vi "Digitizer Analyze_SNRDCOffset.vi"(6 "frequency range":T1={"start frequency"=-1.0, "stop frequency"=-1.0}, 7 "Pins":string[](array[string])=["Xout"], 8 "error in":errorcluster, 9 "Published Data Id":string[](array[string]), 10 "Waveform Data In":waveform(dbl)[](array[waveform])=[{"t0"=timestamp(3637030365.2340937 s since 1904-01-01), "dt"=3.3333333333333334e-08, "Y"=array[5343 elements]}, {"t0"=timestamp(3637030365.2340937 s since 1904-01-01), "dt"=3.3333333333333334e-08, "Y"=array[5343 elements]}], 11 "Semiconductor Module Context":T2) -> (0 "error out":errorcluster, 1 "Frequency (Hz)":dbl format="%.2f", 2 "SNR (dB)":dbl format="%.2f", 3 "Power (dBm)":dbl)   [LabVIEW 2014]
doc: "Example: Measurement Library\n\nRecommended Input Signal: 100 kHz, 2 Vpp, sine wave\n\nDevices Supported: Refer to NI Example Finders\n\nLabVIEW Description:\n\nThis example illustrates fetching scalar measurements from NI-SCOPE, such as period and rise time calculations. \n\nSome common horizontal and vertical parameters are configured for the oscilloscope. The property node is used to set the reference level units, and the low, middle and high reference levels. For more information about measurement library parameters, see the NI-SCOPE VI Reference Help file. \n\nAfter the Read VI is called to acquire a waveform, the Fetch Measurement Stats VI is used to perform the desired scalar measurement analysis on the waveform. NI-SCOPE keeps a history of each measurement's results, which allows it to retrieve the statistics computed over multiple acquisitions. These statistics include the mean, standard deviation, min, max and number of acquisitions used in the statistics. The statistics are updated once per acquisition when the measurement is fetched. The Clear Stats VI clears this history."
uses:
  <vilib>/NI_TestStand_SemiconductorModule/NI_TestStand_Semiconductor_Module.lvlibp/PinMap/General/SemiconductorModuleContext.ctl
  <vilib>/NI_TestStand_SemiconductorModule/NI_TestStand_Semiconductor_Module.lvlibp/PinMap/General/NIInstrumentTypeIDs.ctl
  <vilib>/addons/_NISVFA/_Shared subVIs/Controls/svc_Window.ctl
  <vilib>/measure/madcrms.llb/Basic Averaged DC-RMS for 1 Chan.vi
  <vilib>/addons/_NISVFA/_Baseband FFT/SVFA FFT Spectrum (Complex) (1 Ch).vi
  <vilib>/addons/_NISVFA/_Spectrum Processing/SVFA Unit Conversion (Complex) (1 Ch).vi
  <vilib>/NI_TestStand_SemiconductorModule/NI_TestStand_Semiconductor_Module.lvlibp/PinMap/General/Publish/PublishDataDoubleFunctionalTest.vi
  <vilib>/NI_TestStand_SemiconductorModule/NI_TestStand_Semiconductor_Module.lvlibp
  <vilib>/measure/NI_MAPro.lvlib
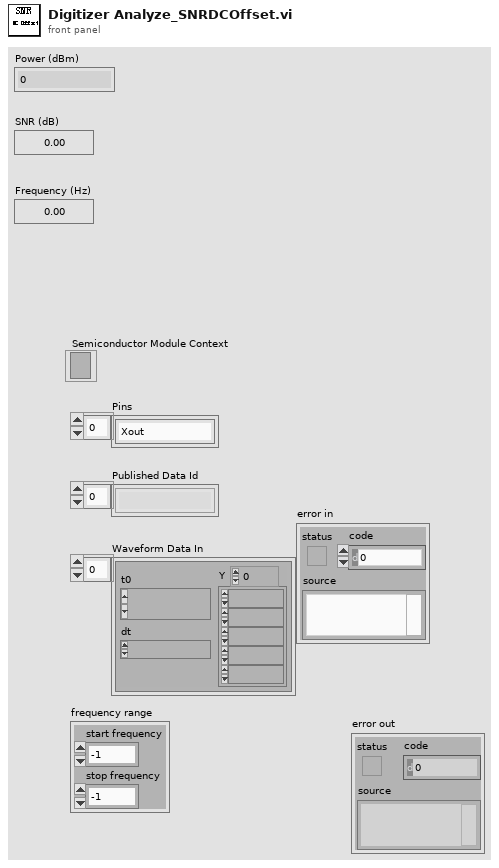
[diagram p1: front panel]
types:
  T1 = cluster{"start frequency":dbl, "stop frequency":dbl}
  T2 = typedef "NI_TestStand_Semiconductor_Module.lvlibp/SemiconductorModuleContext.ctl" = refnum<k7>
  T3 = typedef "svc_Window.ctl" = u32
  T4 = typedef "NI_TestStand_Semiconductor_Module.lvlibp/NIInstrumentTypeIDs.ctl" = string
  T5 = cluster{"linear/dB":enum16{"no change", "linear", "dB"}, "dB reference (0: no change)":dbl, "power/magnitude":enum16{"no change", "power", "magnitude"}, "view":enum16{"no change", "rms", "peak", "peak-peak"}}
  T6 = typedef "svc_Spectrum Info.ctl" = cluster{"channel name":string, "description":string, "x-axis units":T7, "spectral info":cluster{"spectrum type":T8, "linear/dB":enum16{"linear", "dB"}, "window":u16, "window size":i32, "FFT size":i32}, "engineering units":T9, "custom label":string, "dB reference [EU]":dbl, "peak units":enum16{"rms", "peak", "peak-peak"}, "weighting filter":T10, "spectral density?":bool, "unit label":string, "spectrum skewed?":bool, "complimentary spectrum units":T11}
  T7 = typedef "svc_X-Axis Units.ctl" = u16
  T8 = typedef "svc_Spectrum Type.ctl" = enum16{"FFT Spectrum [complex]", "Amplitude [Magnitude]", "Power [Magnitude^2]", "Cross Spectrum [complex]", "Frequency Response [Complex]"}
  T9 = typedef "svc_Engineering Units Text Ring.ctl" = u16
  T10 = typedef "svc_Weighting Filter Text Ring.ctl" = u16
  T11 = typedef "svc_Complimentary Spectrum Units.ctl" = enum16{"none", "radians", "degrees", "cycles", "imaginary"}
  T12 = cluster{"complex spectrum response":cluster{"f0":dbl, "df":dbl, "complex spectrum":cdb[]}, "spectrum info":T6}
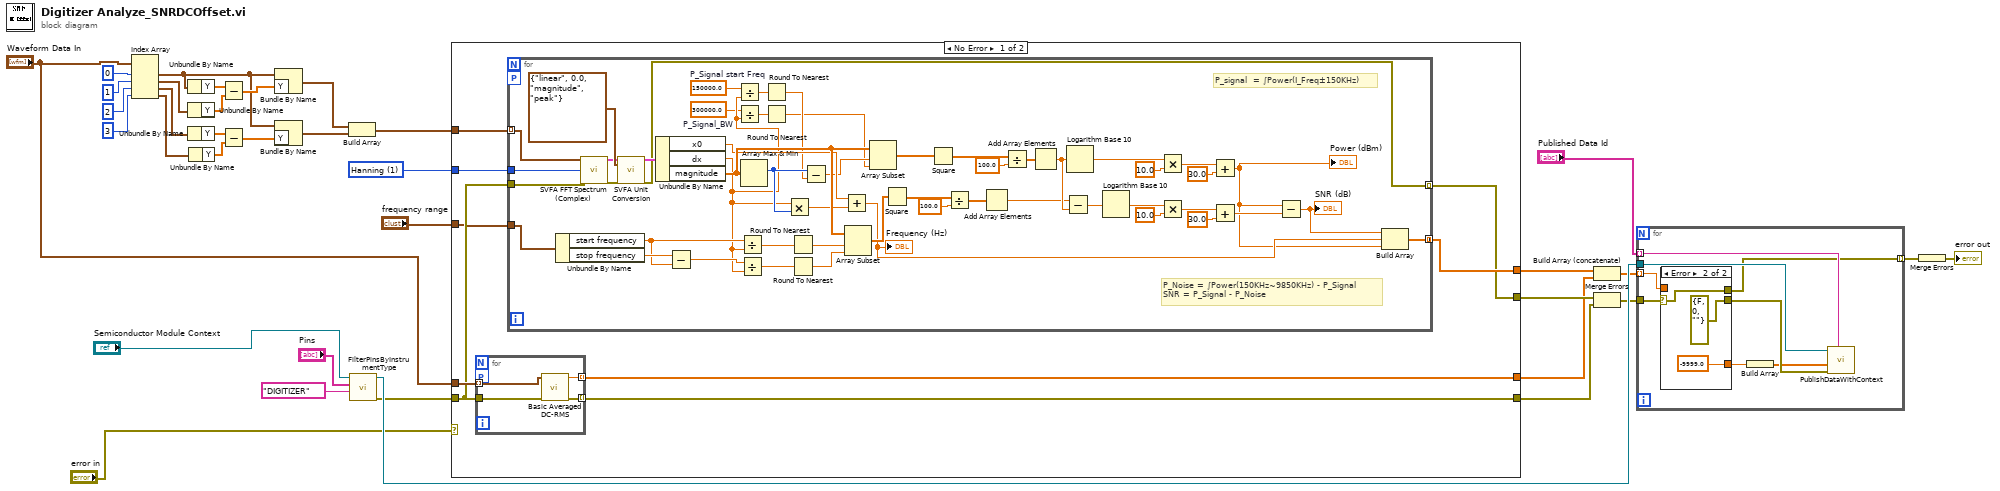
[diagram p0: block diagram]
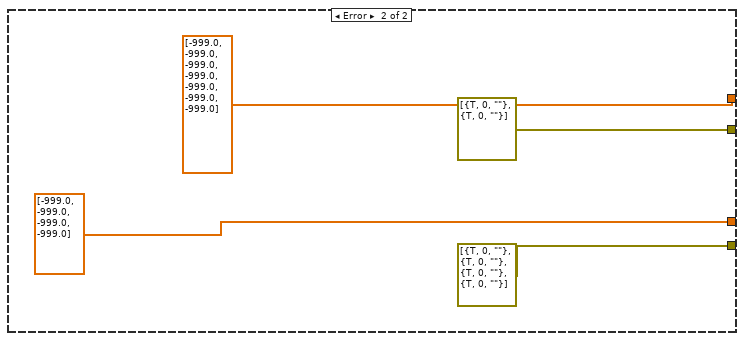
[diagram p2: hidden frame]
diagram:
  w31 = T3 1 items=["None"=0, "Hanning"=1, "Hamming"=2, "Blackman-Harris"=3, "Exact Blackman"=4, "Blackman"=5, "Flat Top"=6, "4 Term B-Harris "=7, "7 Term B-Harris"=8, "Low Sidelobe"=9, "Force"=64, "Exponential"=65, "Blackman Nuttall"=11, "Triangle"=30, "Bartlett-Hanning"=31, "Bohman"=32, "Parzen"=33, "Welch"=34, "Kaiser"=60, "Dolph-Chebyshev"=61, "Gaussian"=62] ("window")
  n1 = Index Array(array="Waveform Data In", index #1=0 ("index"), index #2=1 ("index"), index #3=2 ("index"), index #4=3 ("index")) -> (element #1=w15:waveform(dbl), element #2=w24:waveform(dbl), element #3=w22:waveform(dbl), element #4=w21:waveform(dbl))
  n2 = Unbundle By Name(w15) -> ("Y"=w28:dbl[])
  n3 = Unbundle By Name(w24) -> ("Y"=w27:dbl[])
  n4 = Unbundle By Name(w22) -> ("Y"=w18:dbl[])
  n5 = Unbundle By Name(w21) -> ("Y"=w17:dbl[])
  n6 = Subtract(x=w28, y=w27) -> (x-y=w32:dbl[])
  n7 = Subtract(x=w18, y=w17) -> (x-y=w16:dbl[])
  n8 = Bundle By Name(cluster=w15, "Y"=w32) -> (w14:waveform(dbl))
  n9 = Bundle By Name(cluster=w15, "Y"=w16) -> (w13:waveform(dbl))
  n10 = Build Array(w14, w13) -> (w12:waveform(dbl)[])
  n11 = call <vilib>:"FilterPinsByInstrumentType.vi"("Instrument Type Id"=T4 "DIGITIZER", "Pins"="Pins", "Semiconductor Module Context"="Semiconductor Module Context") -> ("error out"=w6:errorcluster, "Semiconductor Module Context Out"=w25:T2)  [unwired: 6 in, 1 out]
  n12 = case shown="No Error" "error in" {
    tunnel: w31 -> [w36 _]
    tunnel: "frequency range" -> [w37 _]
    tunnel: w12 -> [w41 _]
    tunnel: "Waveform Data In" -> [w44 _]
    tunnel: [w39 dbl[] [-999.0, -999.0, -999.0, -999.0, -999.0, -999.0, -999.0]] -> w8
    tunnel: w6 -> [w40 _]
    tunnel: [w38 errorcluster[] [{"status"=TRUE, "code"=0, "source"=""}, {"status"=TRUE, "code"=0, "source"=""}]] -> w5
    tunnel: [w43 errorcluster[] [{"status"=TRUE, "code"=0, "source"=""}, {"status"=TRUE, "code"=0, "source"=""}, {"status"=TRUE, "code"=0, "source"=""}, {"status"=TRUE, "code"=0, "source"=""}]] -> w4
    tunnel: [w42 dbl[] [-999.0, -999.0, -999.0, -999.0]] -> w2
    frame No Error {
      n13 = for {
        tunnel: w44 -> [w100] mode=indexing
        tunnel: [w97] -> w42 mode=indexing
        tunnel: w40 -> [w99]
        tunnel: [w98] -> w43 mode=indexing
        workers-P: _ -> [_]
        n14 = call-poly <vilib>:"Basic Averaged DC-RMS.vi"("error in (no error)"=w99, "signal in"=w100) -> ("error out"=w98:errorcluster, "DC value"=w97:dbl)  [unwired: 6 in, 2 out]
      }
      n15 = for {
        tunnel: w41 -> [w63] mode=indexing
        tunnel: w36 -> [w64]
        tunnel: [w96] -> w39 mode=concatenating
        tunnel: w37 -> [w59]
        workers-P: _ -> [_]
        tunnel: w40 -> [w65]
        tunnel: [w66] -> w38 mode=indexing
        w47 = 300000.0  # P_Signal_BW
        w48 = 150000.0  # P_Signal start Freq
        # "P_Noise = ∫Power(150KHz~9850KHz) - P_Signal\nSNR = P_Signal - P_Noise"
        # "P_signal  = ∫Power(I_Freq±150KHz)"
        n16 = Unbundle By Name(w59) -> ("start frequency"=w55:dbl, "stop frequency"=w56:dbl)
        n17 = call-poly <vilib>:"SVFA FFT Spectrum (Complex).vi"("scaled signal [EU]"=w63, "window"=w64, "error in"=w65) -> ("complex spectrum"=w67:T12, "error out"=w68:errorcluster)  [unwired: 13 in, 2 out]
        n18 = call-poly <vilib>:"SVFA Unit Conversion.vi"("complex spectrum"=w67, "desired scaling"=T5 {"linear/dB"=enum."linear", "dB reference (0: no change)"=0.0, "power/magnitude"=enum."magnitude", "view"=enum."peak"}, "error in (no error)"=w68) -> ("converted spectrum"=w70:cluster{"x0":dbl, "dx":dbl, "magnitude":dbl[]}, "error out"=w66:errorcluster)  [unwired: 11 in, 4 out]
        n19 = Unbundle By Name(w70) -> ("x0"=w80:dbl, "dx"=w49:dbl, "magnitude"=w83:dbl[])
        n20 = Subtract(x=w56, y=w55) -> (x-y=w54:dbl)
        n21 = Divide(x=w48, y=w49) -> (x/y=w51:dbl)
        n22 = Divide(x=w47, y=w49) -> (x/y=w50:dbl)
        n23 = Divide(x=w55, y=w49) -> (x/y=w58:dbl)
        n24 = Divide(x=w54, y=w49) -> (x/y=w53:dbl)
        n25 = Array Max & Min(array=w83) -> (max index (indices)=w82:i32)  [unwired: 3 out]
        n26 = Round To Nearest(number=w51) -> (nearest integer value=w46:dbl)
        n27 = Round To Nearest(number=w50) -> (nearest integer value=w45:dbl)
        n28 = Multiply(x=w49, y=w82) -> (x*y=w81:dbl)
        n29 = Round To Nearest(number=w58) -> (nearest integer value=w57:dbl)
        n30 = Round To Nearest(number=w53) -> (nearest integer value=w52:dbl)
        n31 = Subtract(x=w82, y=w46) -> (x-y=w71:dbl)
        n32 = Add(x=w80, y=w81) -> (x+y=w61:dbl)
        "Frequency (Hz)" <- w61
        n33 = Array Subset(array=w83, index=w57, length=w52) -> (w91:dbl[])
        n34 = Array Subset(array=w83, index=w71, length=w45) -> (w72:dbl[])
        n35 = Square(x=w91) -> (x^2=w84:dbl[])
        n36 = Square(x=w72) -> (x^2=w73:dbl[])
        n37 = Divide(x=w84, y=100.0) -> (x/y=w86:dbl[])
        n38 = Add Array Elements(numeric array=w86) -> (sum=w92:dbl)
        n39 = Divide(x=w73, y=100.0) -> (x/y=w75:dbl[])
        n40 = Add Array Elements(numeric array=w75) -> (sum=w93:dbl)
        n41 = Subtract(x=w92, y=w93) -> (x-y=w94:dbl)
        n42 = Logarithm Base 10(1:w93) -> (0:w76:dbl)
        n43 = Logarithm Base 10(1:w94) -> (0:w87:dbl)
        n44 = Multiply(x=w76, y=10.0) -> (x*y=w78:dbl)
        n45 = Multiply(x=w87, y=10.0) -> (x*y=w89:dbl)
        n46 = Add(x=w78, y=30.0) -> (x+y=w60:dbl)
        "Power (dBm)" <- w60
        n47 = Add(x=w89, y=30.0) -> (x+y=w95:dbl)
        n48 = Subtract(x=w60, y=w95) -> (x-y=w62:dbl)
        "SNR (dB)" <- w62
        n49 = Build Array(w62, w61, w60) -> (w96:dbl[])
      }
    }
    frame Error {
    }
  }
  n50 = Build Array (concatenate)(w8, w2) -> (w7:dbl[])
  n51 = Merge Errors(w5, w4) -> (w3:errorcluster)
  n52 = for {
    tunnel: "Published Data Id" -> [w112] mode=indexing
    tunnel: w7 -> [w109] mode=indexing
    tunnel: w25 -> [w111]
    tunnel: w3 -> [w110]
    tunnel: [w106] -> w11 mode=indexing
    n53 = case shown="Error" w110 {
      selector: w110 -> [w113 w116]
      tunnel: w109 -> [w114 _]
      tunnel: [w114 -9999.0 ("detected fundamental\nfrequency [Hz]")] -> w108
      tunnel: [w113 errorcluster {"status"=FALSE, "code"=0, "source"=""} ("error IO")] -> w107
      tunnel: [w113 w116] -> w106
      frame No Error {
      }
      frame Error {
      }
    }
    n54 = Build Array(w108) -> (w105:dbl[])
    n55 = call-poly <vilib>:"PublishDataWithContext.vi"("Published Data Id"=w112, "error in (no error)"=w107, "Data In"=w105, "Semiconductor Module Context"=w111) -> ()  [unwired: 6 in, 2 out]
  }
  n56 = Merge Errors(w11) -> (→"error out":errorcluster)
